vi "Interpolate Linear.vi"(9 "X in":dbl[](array[numeric]), 10 "Y in":dbl[](array[numeric])) -> (2 "yi":dbl[](array[numeric]) format="%_6g")   [LabVIEW 2014]
uses:
  <vilib>/gmath/NI_Gmath.lvlib
panel:
  out "X in 2":dbl[](array[numeric])
  out "Y in 2":dbl[](array[numeric])
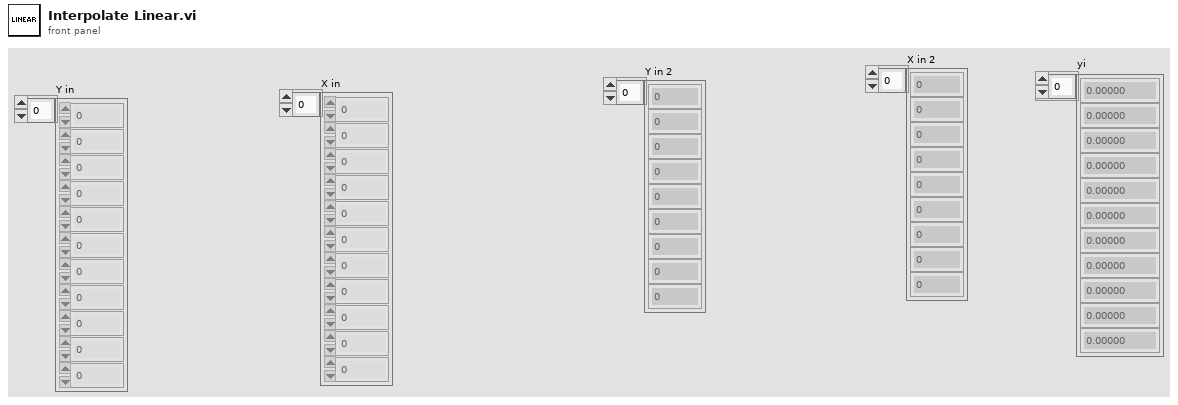
[diagram p1: front panel]
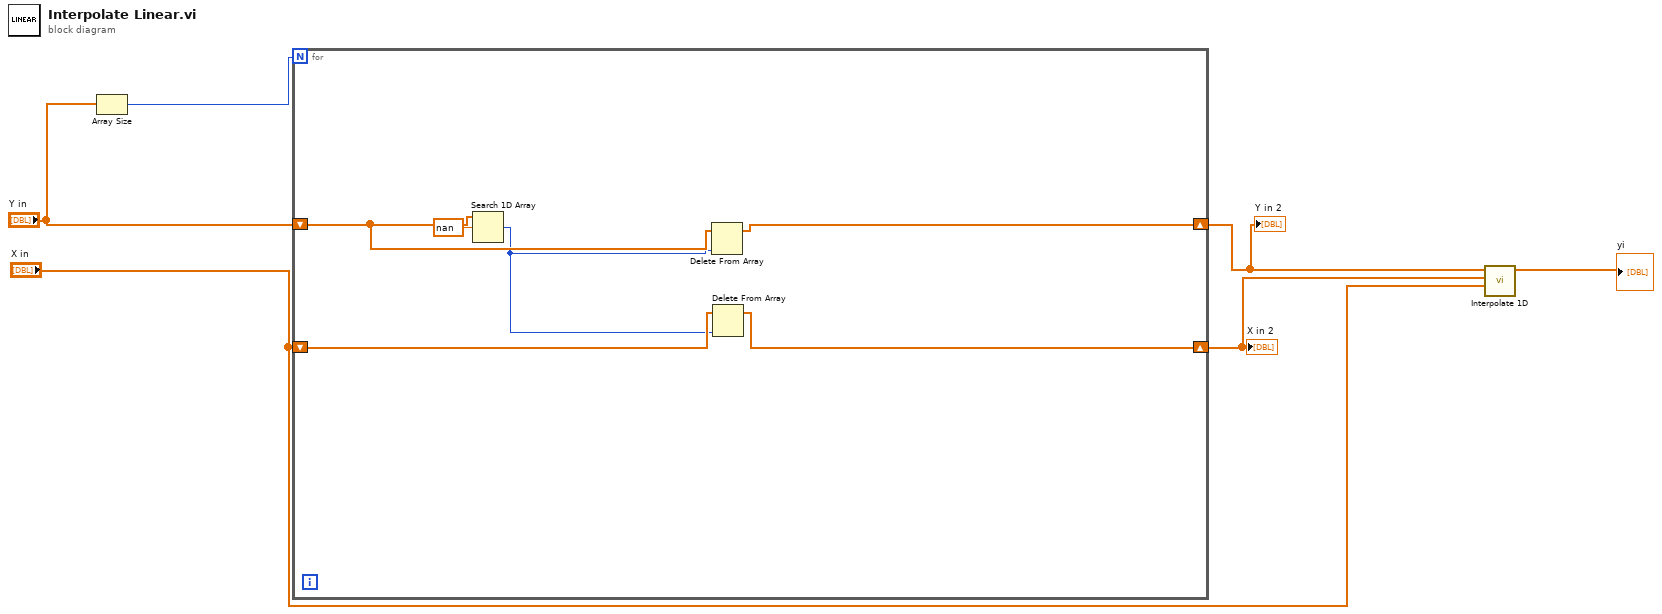
[diagram p0: block diagram]
diagram:
  n1 = Array Size(array="Y in") -> (size(s)=w6:i32)
  n2 = for {
    N: w6 -> [_]
    shift-right: [w8] -> w4
    shift-left: "Y in" -> [w11]
    shift-right: [w7] -> w3
    shift-left: "X in" -> [w10]
    n3 = Search 1D Array(1D array=w11, element=nan) -> (index of element=w9:i32)  [unwired: 1 in]
    n4 = Delete From Array(array=w11, index=w9) -> (array with subset deleted=w8:dbl[])  [unwired: 1 in, 1 out]
    n5 = Delete From Array(array=w10, index=w9) -> (array with subset deleted=w7:dbl[])  [unwired: 1 in, 1 out]
  }
  "Y in 2" <- w4
  "X in 2" <- w3
  n6 = call <vilib>:"Interpolate 1D.vi"("xi"="X in", "X"=w3, "Y"=w4) -> ("yi"=→"yi":dbl[])  [unwired: 6 in, 2 out]
